vi "FezDuck.vi"() -> ()   [LabVIEW 2021]
uses:
  Control 1.ctl
panel:
  out "Output 2":dbl(knob) scale=0.0..750.0
  in  "D":dbl(knob) scale=0.0..10.0
  in  "C":dbl(knob) scale=0.0..10.0
  in  "B":dbl(knob) scale=0.0..10.0
  in  "A":dbl(knob) min=0.0 max=10.0 step=1.0 scale=0.0..10.0
  in  "Combo Box":T1
  out "Output":dbl
  in  "Num2":dbl
  in  "num1":dbl
  # "."
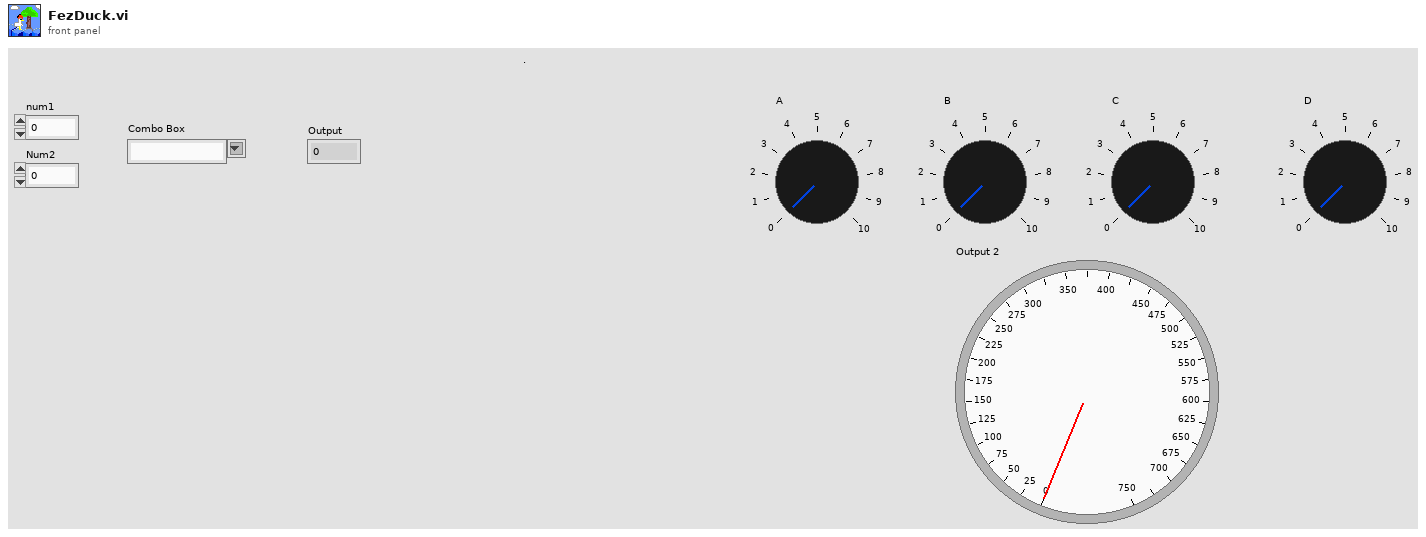
[diagram p1: front panel]
types:
  T1 = typedef "Control 1.ctl" = string
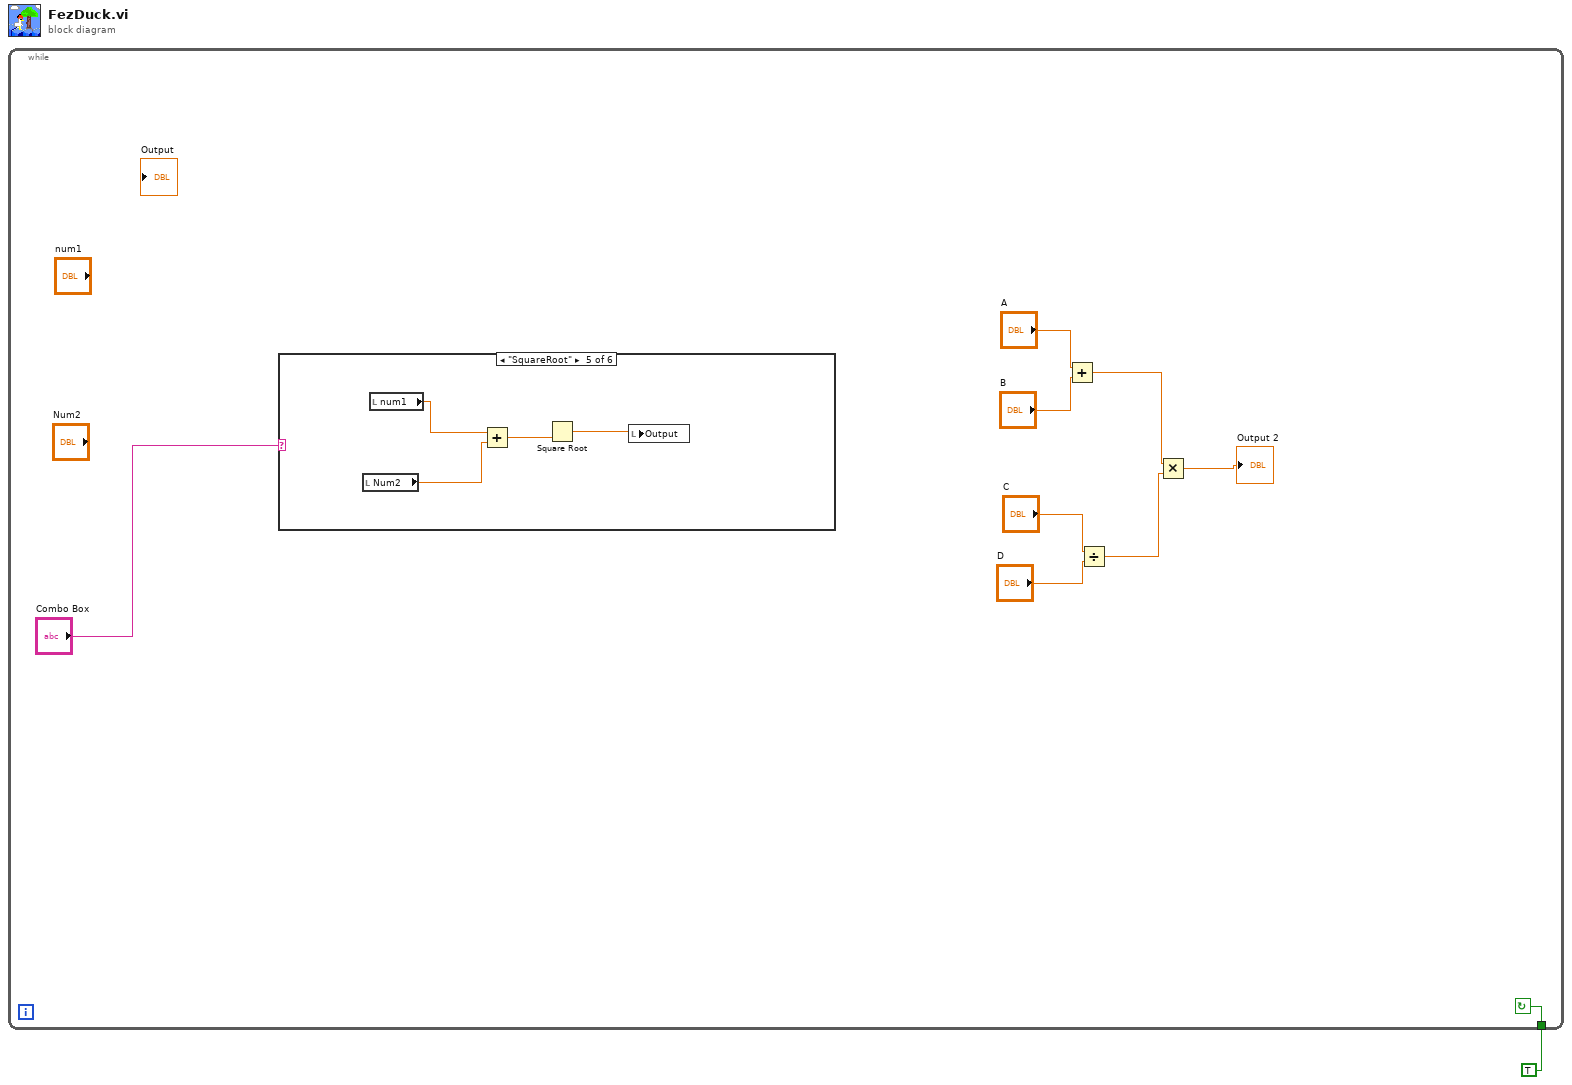
[diagram p0: block diagram]
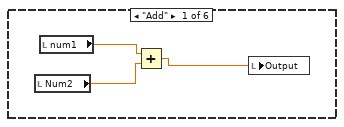
[diagram p2: hidden frame]
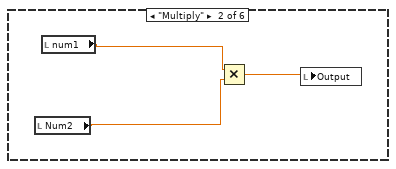
[diagram p3: hidden frame]
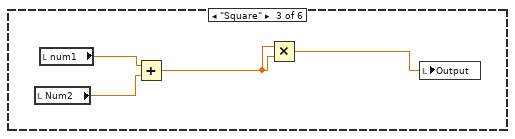
[diagram p4: hidden frame]
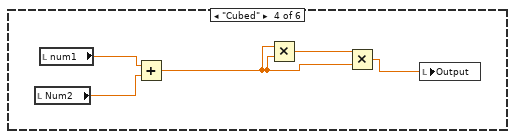
[diagram p5: hidden frame]
diagram:
  n1 = while {
    tunnel: TRUE -> [w10]
    stop <- w10 continue-if-true
    n2 = case shown="\"SquareRoot\"" "Combo Box" {
      frame "Add" {
        n3 = local read "Num2"() -> (w12:dbl)
        n4 = local read "num1"() -> (w13:dbl)
        n5 = Add(x=w13, y=w12) -> (x+y=w11:dbl)
        n6 = local write "Output"(w11) -> ()
      }
      frame "Multiply" {
        n7 = local read "Num2"() -> (w15:dbl)
        n8 = local read "num1"() -> (w14:dbl)
        n9 = Multiply(x=w14, y=w15) -> (x*y=w16:dbl)
        n10 = local write "Output"(w16) -> ()
      }
      frame "Square" {
        n11 = local read "Num2"() -> (w18:dbl)
        n12 = local read "num1"() -> (w17:dbl)
        n13 = Add(x=w17, y=w18) -> (x+y=w19:dbl)
        n14 = Multiply(x=w19, y=w19) -> (x*y=w20:dbl)
        n15 = local write "Output"(w20) -> ()
      }
      frame "Cubed" {
        n16 = local read "Num2"() -> (w22:dbl)
        n17 = local read "num1"() -> (w21:dbl)
        n18 = Add(x=w21, y=w22) -> (x+y=w25:dbl)
        n19 = Multiply(x=w25, y=w25) -> (x*y=w23:dbl)
        n20 = Multiply(x=w23, y=w25) -> (x*y=w24:dbl)
        n21 = local write "Output"(w24) -> ()
      }
      frame "SquareRoot" {
        n22 = local read "Num2"() -> (w27:dbl)
        n23 = local read "num1"() -> (w28:dbl)
        n24 = Add(x=w28, y=w27) -> (x+y=w29:dbl)
        n25 = Square Root(x=w29) -> (sqrt(x)=w26:dbl)
        n26 = local write "Output"(w26) -> ()
      }
      frame Default {
      }
    }
    n27 = Add(x="A", y="B") -> (x+y=w4:dbl)
    n28 = Divide(x="C", y="D") -> (x/y=w5:dbl)
    n29 = Multiply(x=w4, y=w5) -> (x*y=→"Output 2":dbl)
  }
